vi "RQST Lookup Table.vi"(7 "Action":T3, 8 "error in (no error)":errorcluster, 9 "ID":u32, 10 "Data":T2, 11 "Rqst LUT":T1) -> (0 "error out":errorcluster, 1 "Found?":bool, 2 "Data Out":T2, 3 "Rqst LUT out":T1)   [LabVIEW 2015, in "J1939 Addon Engine.lvlib"]
uses:
  Engine/J1939 Addon Engine.lvlib
  Types/RQST Lookup Table Cluster.ctl
  <vilib>/xnet/xnet.llb/XNET Frame CAN.ctl
  <vilib>/xnet/xnet.llb/XNET Frame Type CAN.ctl
  Types/RQST Lookup Table Action.ctl
  Types/RQST Lookup Table Reference.ctl
panel:
  # "OUTPUTS"
  # "INPUTS"
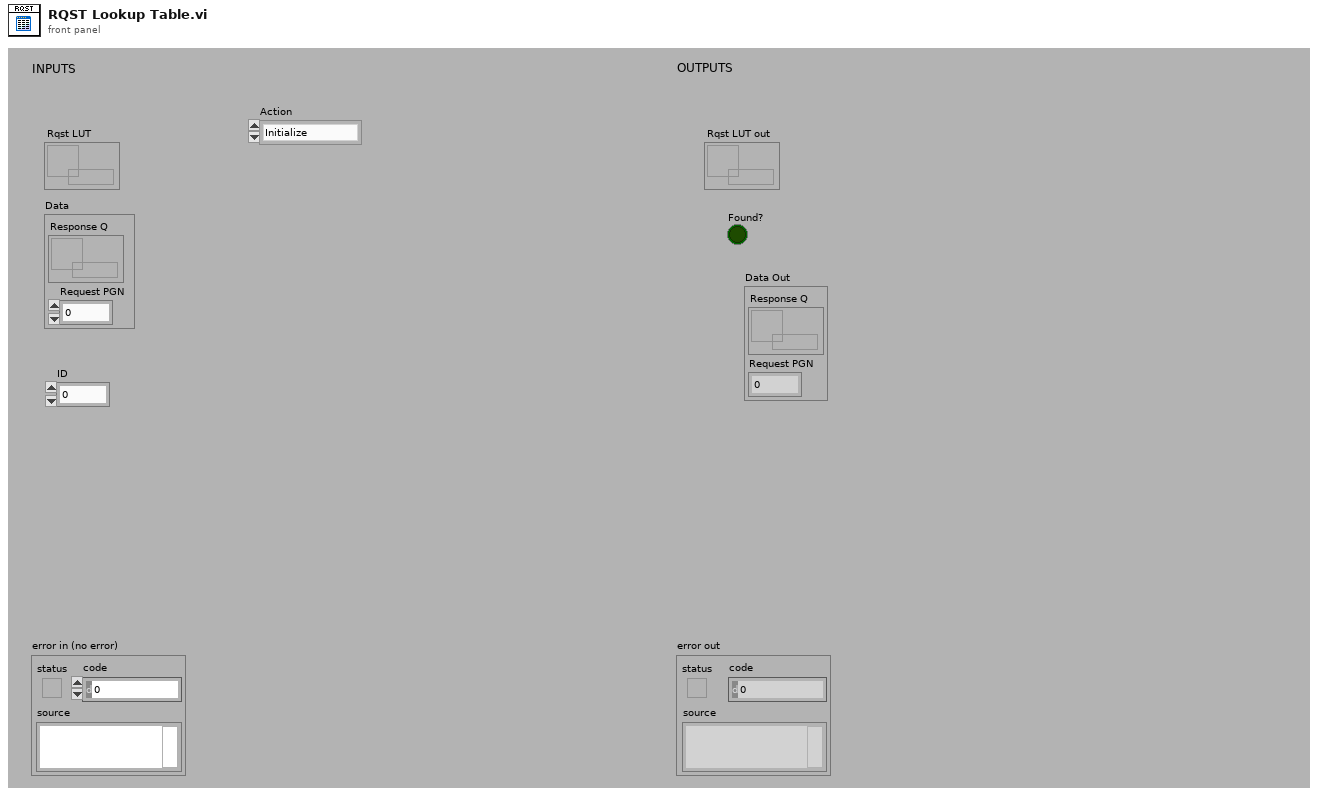
[diagram p1: front panel]
types:
  T1 = typedef "J1939 Addon Engine.lvlib/RQST Lookup Table Reference.ctl" = refnum<data-value>
  T2 = typedef "J1939 Addon Engine.lvlib/RQST Lookup Table Cluster.ctl" = cluster{"Response Q":refnum<queue>, "Request PGN":u32}
  T3 = typedef "J1939 Addon Engine.lvlib/RQST Lookup Table Action.ctl" = enum16{"Initialize", "Add", "Get", "Remove"}
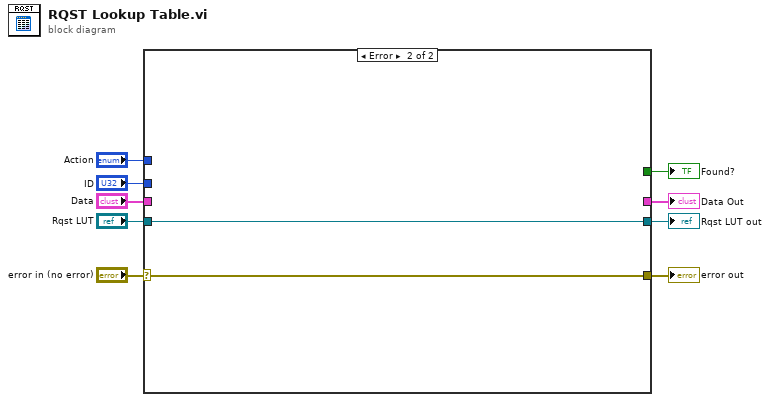
[diagram p0: block diagram]
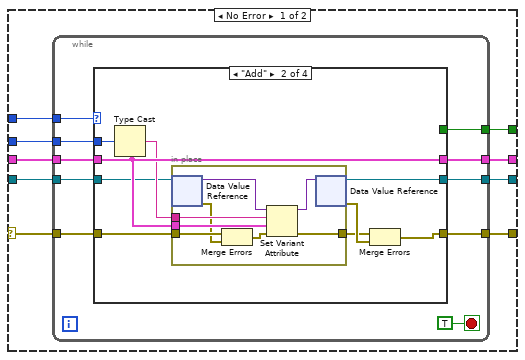
[diagram p2: hidden frame]
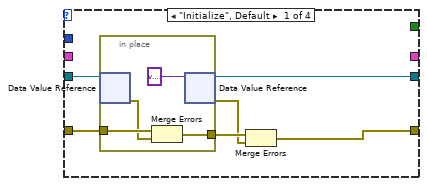
[diagram p3: hidden frame]
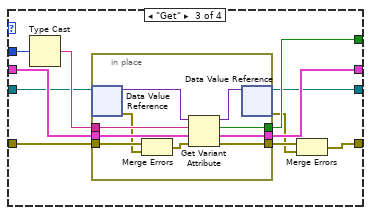
[diagram p4: hidden frame]
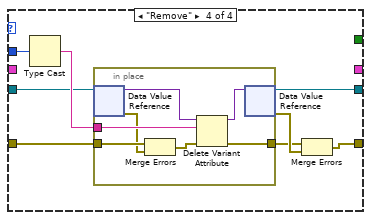
[diagram p5: hidden frame]
diagram:
  n1 = case shown="Error" "error in (no error)" {
    selector: "error in (no error)" -> [w14 w93]
    tunnel: [w13 w93] -> w8
    tunnel: "Data" -> [w17 _]
    tunnel: "Action" -> [w18 _]
    tunnel: [w16 _] -> w5
    tunnel: "ID" -> [w15 _]
    tunnel: [w12 _] -> w3
    tunnel: "Rqst LUT" -> [w11 w92]
    tunnel: [w10 w92] -> w1
    frame No Error {
      n2 = while {
        tunnel: w18 -> [w28]
        tunnel: w17 -> [w27]
        tunnel: [w25] -> w16
        tunnel: w15 -> [w24]
        tunnel: w14 -> [w23]
        tunnel: [w22] -> w13
        tunnel: [w21] -> w12
        tunnel: w11 -> [w20]
        tunnel: [w19] -> w10
        stop <- TRUE stop-if-true
        n3 = case shown="\"Add\"" w28 {
          tunnel: w27 -> [_ w47 w62 _]
          tunnel: [_ w47 w61 _] -> w25
          tunnel: w24 -> [_ w46 w66 w84]
          tunnel: w23 -> [w32 w44 w64 w83]
          tunnel: [w29 w40 w58 w78] -> w22
          tunnel: [_ _ w60 _] -> w21
          tunnel: w20 -> [w34 w43 w59 w81]
          tunnel: [w33 w42 w56 w80] -> w19
          frame "Initialize", Default {
            n4 = in-place {
              in-place-border: w32 -> [w37]
              in-place-border: [w35] -> w31
              n5 = in-place-dvr #1(w34) -> (w36:errorcluster)  [unwired: 1 out]
              n6 = Merge Errors(w37, w36) -> (w35:errorcluster)
              n7 = in-place-dvr #1(variant ("duplicate variant")) -> (w33:T1, w30:errorcluster)
            }
            n8 = Merge Errors(w31, w30) -> (w29:errorcluster)
          }
          frame "Add" {
            n9 = Type Cast(x=w46) -> (*(type *) &x=w45:string)  [unwired: 1 in]
            n10 = in-place {
              in-place-border: w47 -> [w55]
              in-place-border: w45 -> [w54]
              in-place-border: w44 -> [w53]
              in-place-border: [w52] -> w39
              n11 = in-place-dvr #2(w43) -> (w51:variant, w48:errorcluster)
              n12 = Merge Errors(w53, w48) -> (w49:errorcluster)
              n13 = Set Variant Attribute(Variant=w51, name=w54, value=w55, error in=w49) -> (Variant out=w50:variant, error out=w52:errorcluster)  [unwired: 1 out]
              n14 = in-place-dvr #2(w50) -> (w42:T1, w41:errorcluster)
            }
            n15 = Merge Errors(w39, w41) -> (w40:errorcluster)
          }
          frame "Get" {
            n16 = Type Cast(x=w66) -> (*(type *) &x=w65:string)  [unwired: 1 in]
            n17 = in-place {
              in-place-border: w65 -> [w76]
              in-place-border: w64 -> [w75]
              in-place-border: [w74] -> w63
              in-place-border: w62 -> [w73]
              in-place-border: [w72] -> w61
              in-place-border: [w71] -> w60
              n18 = in-place-dvr #3(w59) -> (w70:variant, w67:errorcluster)
              n19 = Merge Errors(w75, w67) -> (w68:errorcluster)
              n20 = Get Variant Attribute(Variant=w70, name=w76, default value (empty Variant)=w73, error in=w68) -> (duplicate Variant=w69:variant, found=w71:bool, value=w72:T2, error out=w74:errorcluster)
              n21 = in-place-dvr #3(w69) -> (w56:T1, w57:errorcluster)
            }
            n22 = Merge Errors(w63, w57) -> (w58:errorcluster)
          }
          frame "Remove" {
            n23 = Type Cast(x=w84) -> (*(type *) &x=w82:string)  [unwired: 1 in]
            n24 = in-place {
              in-place-border: w83 -> [w91]
              in-place-border: [w90] -> w77
              in-place-border: w82 -> [w89]
              n25 = in-place-dvr #4(w81) -> (w88:variant, w86:errorcluster)
              n26 = Merge Errors(w91, w86) -> (w87:errorcluster)
              n27 = Delete Variant Attribute(4:w87, 6:w89, 7:w88) -> (0:w90:errorcluster, 3:w85:variant)  [unwired: 1 out]
              n28 = in-place-dvr #4(w85) -> (w80:T1, w79:errorcluster)
            }
            n29 = Merge Errors(w77, w79) -> (w78:errorcluster)
          }
        }
      }
    }
    frame Error {
    }
  }
  "error out" <- w8
  "Data Out" <- w5
  "Found?" <- w3
  "Rqst LUT out" <- w1
